vi "Session.CheckValid.vi"(10 "Cached Session":T1, 11 "requested session":T1) -> (2 "Error Code":i32, 3 "Valid?":bool)   [LabVIEW 2025, in "bus_monitor_server_do.lvlib"]
doc: "Check that the requested session matches the current running session AND is NOT empty."
uses:
  bus_monitor_server_do.lvlib
  bus_monitor_server/RPC Messages/ni_bus_monitor_api_Session.ctl
  bus_monitor_server/bus_monitor_server.lvlib
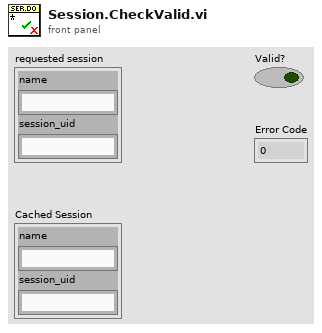
[diagram p1: front panel]
types:
  T1 = typedef "bus_monitor_server.lvlib/ni_bus_monitor_api_Session.ctl" = cluster{"name":string, "session_uid":string}
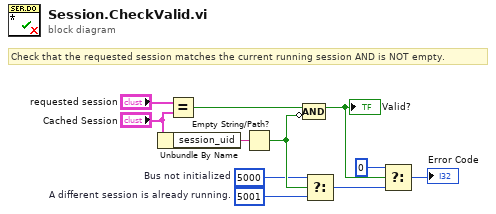
[diagram p0: block diagram]
diagram:
  w5 = 5001  # A different session is already running.
  w6 = 5000  # Bus not initialized
  # "Check that the requested session matches the current running session AND is NOT empty."
  n1 = Unbundle By Name("Cached Session") -> ("session_uid"=w8:string)
  n2 = Equal?(x="requested session", y="Cached Session") -> (x = y?=w11:bool)
  n3 = Empty String/Path?(string/path=w8) -> (empty?=w7:bool)
  n4 = Compound Arithmetic op=AND(w11, invert w7) -> (w4:bool)
  "Valid?" <- w4
  n5 = Select(t=w6, s=w7, f=w5) -> (s? t:f=w3:i32)
  n6 = Select(t=0, s=w4, f=w3) -> (s? t:f=→"Error Code":i32)
